vi "Mexa_One.vi"(0 "String 1 In":string, 1 "Connect":bool, 5 "connection ID 1 In":refnum<k5>, 7 "error out 1 In":errorcluster, 9 "connection ID 2 In":refnum<k16>, 11 "error out 2 In":errorcluster, 12 "Time In":i16, 13 "Test Loop":dbl) -> (3 "Emissions":dbl[](array[numeric]), 4 "String 1 Out":string, 6 "connection ID 1 Out":refnum<k5>, 8 "error 1 out":errorcluster, 10 "connection ID 2 Out":refnum<k16>, 14 "Time Out":i16, 15 "error 2 out":errorcluster)   [LabVIEW 2014]
panel:
  in  "stop":bool
  out "Array out":dbl[](array[numeric])
  in  "stop TCP 2":bool
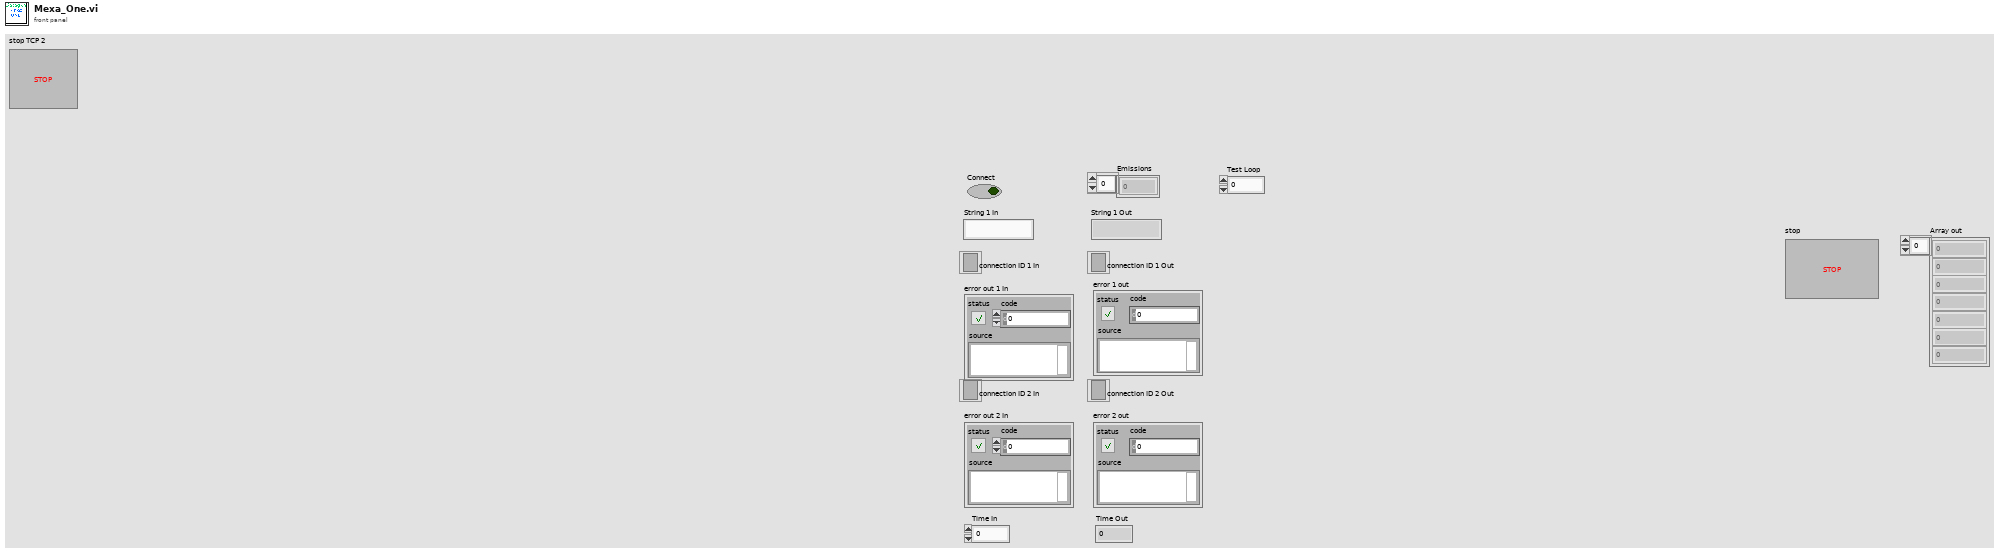
[diagram p1: front panel]
types:
  T1 = cluster{"status":bool, "code":bool, "source":bool}
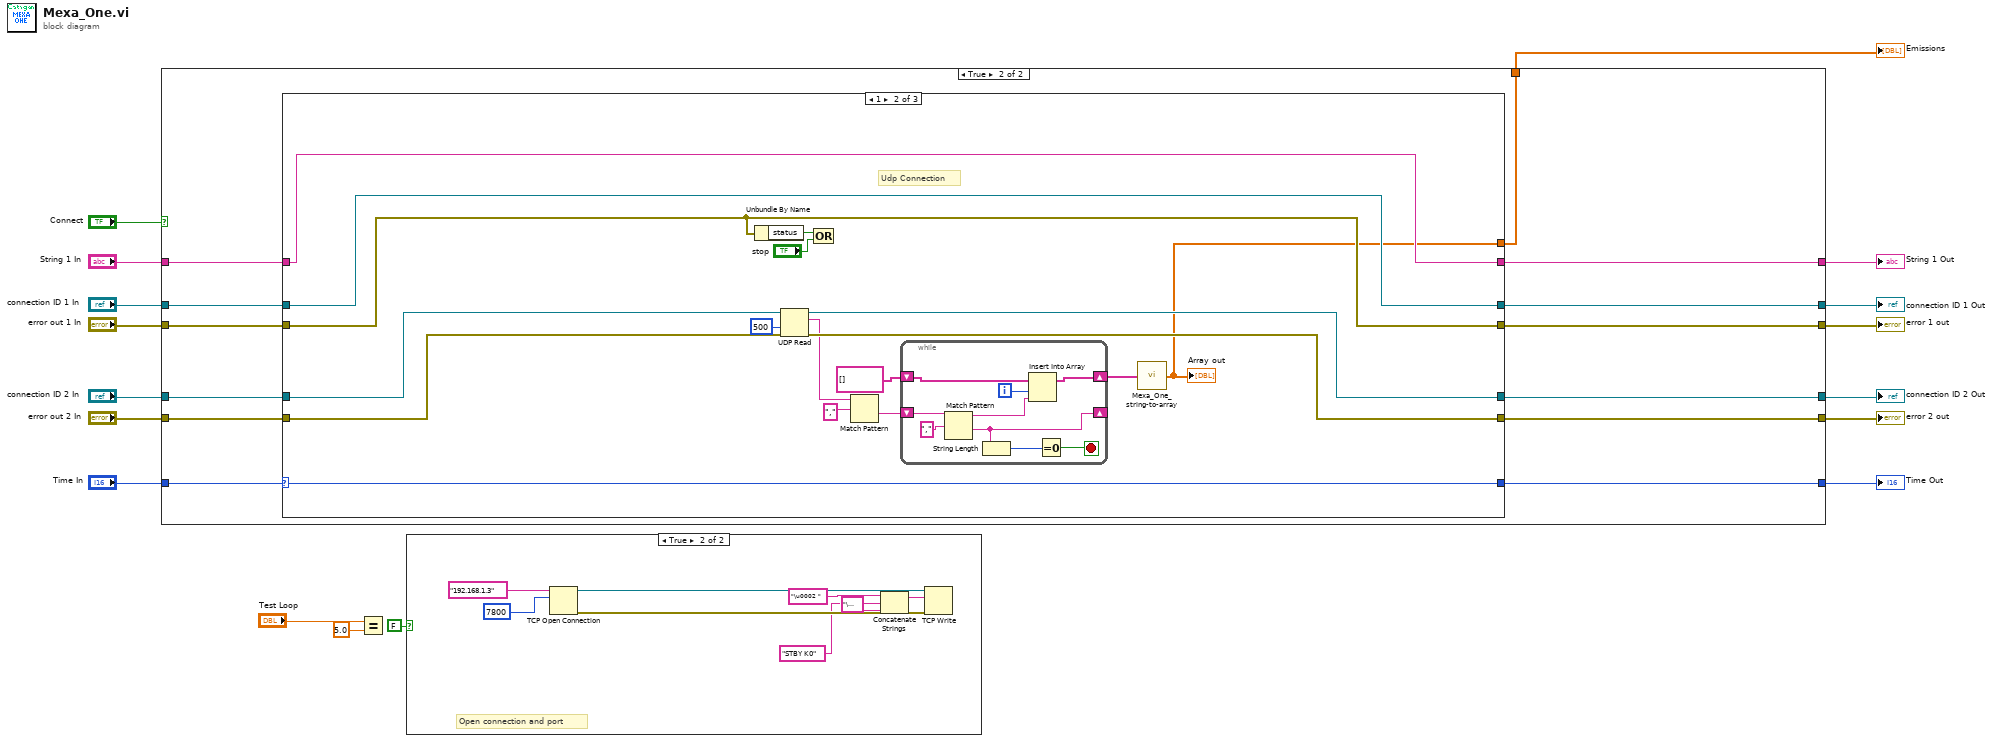
[diagram p0: block diagram]
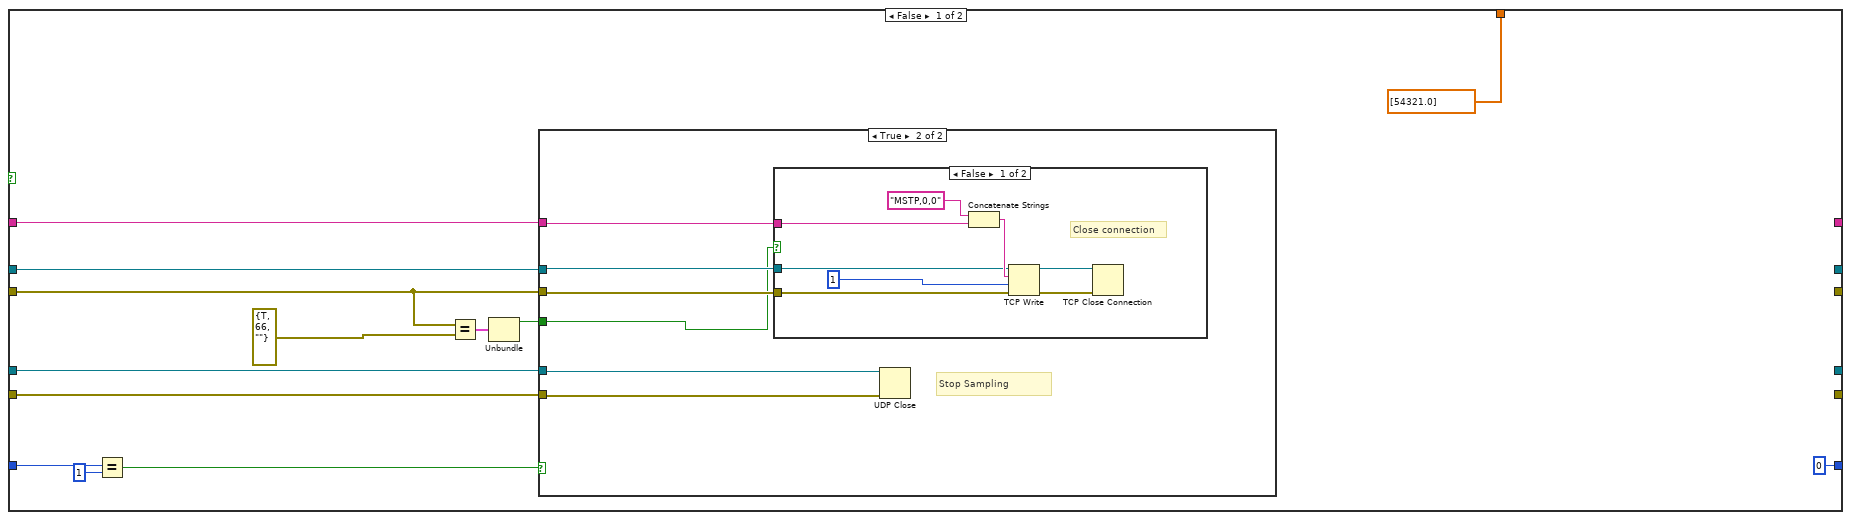
[diagram p3: hidden frame]
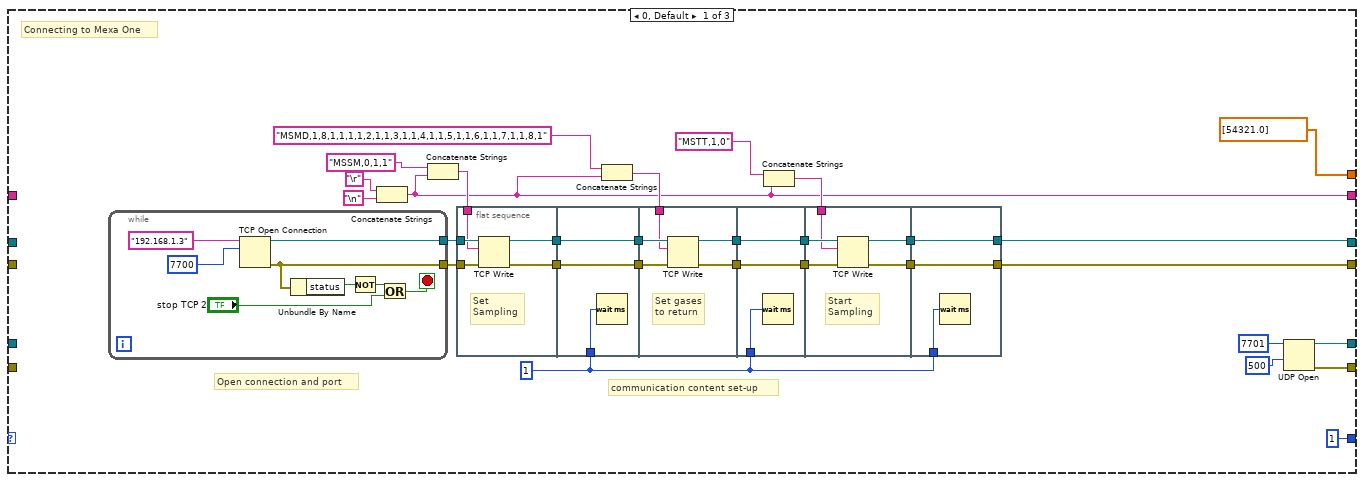
[diagram p6: hidden frame]
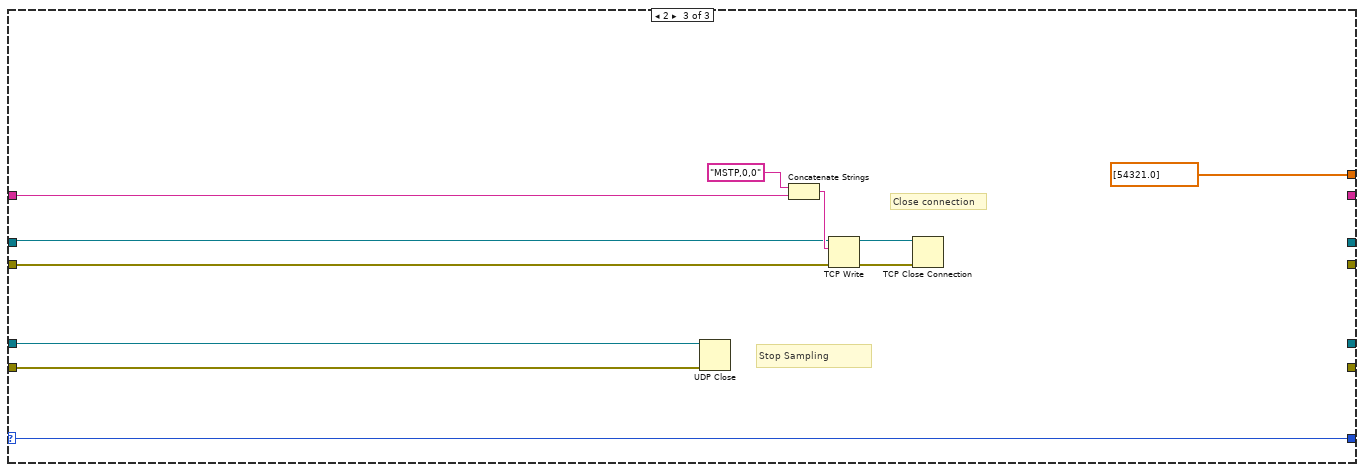
[diagram p7: hidden frame]
diagram:
  n1 = case shown="True" "Connect" {
    tunnel: [dbl[] [54321.0] w57] -> w4
    tunnel: [_ w56] -> w6
    tunnel: [_ w55] -> w7
    tunnel: "connection ID 1 In" -> [w24 w54]
    tunnel: "error out 1 In" -> [w21 w53]
    tunnel: [_ w52] -> w5
    tunnel: "String 1 In" -> [w25 w51]
    tunnel: [_ w50] -> w8
    tunnel: [_ w49] -> w9
    tunnel: "connection ID 2 In" -> [w23 w48]
    tunnel: "error out 2 In" -> [w22 w47]
    tunnel: "Time In" -> [w28 w46]
    tunnel: [i16 0 ("MKS 2") w45] -> w10
    frame False {
      n2 = Equal?(x=w28, y=i16 1) -> (x = y?=w26:bool)
      n3 = Equal?(x=w21, y=errorcluster {"status"=TRUE, "code"=66, "source"=""}) -> (x = y?=w19:T1)
      n4 = Unbundle(w19) -> ("status"=w18:bool)  [unwired: 2 out]
      n5 = case shown="True" w26 {
        tunnel: w25 -> [_ w36]
        tunnel: w24 -> [_ w32]
        tunnel: w21 -> [_ w33]
        tunnel: w23 -> [_ w35]
        tunnel: w22 -> [_ w34]
        tunnel: w18 -> [_ w31]
        frame False {
        }
        frame True {
          # "Stop Sampling"
          n6 = case shown="False" w31 {
            tunnel: w36 -> [w40 _]
            tunnel: w33 -> [w39 _]
            tunnel: w32 -> [w38 _]
            frame False {
              # "Close connection"
              n7 = Concatenate Strings("MSTP,0,0" ("string"), w40) -> (w41:string)
              n8 = TCP Write(connection ID=w38, data in=w41, error in (no error)=w39, 9:1 ("timeout ms (25000)")) -> (connection ID out=w43:refnum<k5>, error out=w44:errorcluster)  [unwired: 1 out]
              n9 = TCP Close Connection(connection ID=w43, error in (no error)=w44) -> ()  [unwired: 1 in, 2 out]
            }
            frame True {
            }
          }
          n10 = UDP Close(connection ID=w35, 8:w34) -> ()  [unwired: 2 out]
        }
      }
    }
    frame True {
      n11 = case shown="1" w46 {
        selector: w46 -> [_ w122 w147]
        tunnel: [dbl[] [54321.0] w120 dbl[] [54321.0]] -> w57
        tunnel: [w65 w135 _] -> w56
        tunnel: [w64 w134 _] -> w55
        tunnel: w54 -> [_ w135 w152]
        tunnel: w53 -> [_ w134 w151]
        tunnel: [w63 w136 _] -> w52
        tunnel: w51 -> [_ w136 w146]
        tunnel: [w60 w131 _] -> w50
        tunnel: [w59 w130 _] -> w49
        tunnel: w48 -> [_ w133 w150]
        tunnel: w47 -> [_ w132 w149]
        tunnel: [i16 1 ("MKS 2") w122 w147] -> w45
        frame 0, Default {
          w66 = 1
          # "Open connection and port"
          # "communication content set-up"
          # "Connecting to Mexa One"
          n12 = while {
            tunnel: [w116] -> w76
            tunnel: [w115] -> w75
            stop <- w112 stop-if-true
            n13 = TCP Open Connection(address="192.168.1.3", remote port or service name=u16 7700) -> (connection ID=w116:refnum<k5>, error out=w115:errorcluster)  [unwired: 3 in]
            n14 = Unbundle By Name(w115) -> ("status"=w117:bool)
            n15 = Not(x=w117) -> (.not. x?=w113:bool)
            n16 = Or(x=w113, y="stop TCP 2") -> (x .or. y?=w112:bool)
          }
          n17 = Concatenate Strings("\r", "\n") -> (w63:string)
          n18 = Concatenate Strings("MSSM,0,1,1" ("data in"), w63) -> (w71:string)
          n19 = flat-sequence {
            tunnel: w76 -> [w92]
            tunnel: w75 -> [w91]
            tunnel: w71 -> [w90]
            tunnel: [w89] -> w86
            tunnel: [w88] -> w85
            tunnel: w86 -> [w95]
            tunnel: w85 -> [w94]
            tunnel: w66 -> [w93]
            tunnel: [w95] -> w84
            tunnel: [w94] -> w83
            tunnel: w84 -> [w99]
            tunnel: w83 -> [w100]
            tunnel: w68 -> [w98]
            tunnel: [w96] -> w82
            tunnel: [w97] -> w81
            tunnel: w82 -> [w103]
            tunnel: w81 -> [w102]
            tunnel: w66 -> [w101]
            tunnel: [w103] -> w80
            tunnel: [w102] -> w79
            tunnel: w80 -> [w107]
            tunnel: w79 -> [w108]
            tunnel: w67 -> [w104]
            tunnel: [w106] -> w78
            tunnel: [w105] -> w77
            tunnel: [w110] -> w65
            tunnel: [w111] -> w64
            tunnel: w78 -> [w111]
            tunnel: w77 -> [w110]
            tunnel: w66 -> [w109]
            frame #0 {
              # "Set \nSampling"
              n20 = TCP Write(connection ID=w92, data in=w90, error in (no error)=w91) -> (connection ID out=w88:refnum<k5>, error out=w89:errorcluster)  [unwired: 1 in, 1 out]
            }
            frame #1 {
              n21 = Wait (ms)(milliseconds to wait=w93) -> ()  [unwired: 1 out]
            }
            frame #2 {
              # "Set gases\nto return"
              n22 = TCP Write(connection ID=w100, data in=w98, error in (no error)=w99) -> (connection ID out=w97:refnum<k5>, error out=w96:errorcluster)  [unwired: 1 in, 1 out]
            }
            frame #3 {
              n23 = Wait (ms)(milliseconds to wait=w101) -> ()  [unwired: 1 out]
            }
            frame #4 {
              # "Start\nSampling"
              n24 = TCP Write(connection ID=w108, data in=w104, error in (no error)=w107) -> (connection ID out=w105:refnum<k5>, error out=w106:errorcluster)  [unwired: 1 in, 1 out]
            }
            frame #5 {
              n25 = Wait (ms)(milliseconds to wait=w109) -> ()  [unwired: 1 out]
            }
          }
          n26 = Concatenate Strings("MSMD,1,8,1,1,1,1,2,1,1,3,1,1,4,1,1,5,1,1,6,1,1,7,1,1,8,1" ("data in"), w63) -> (w68:string)
          n27 = Concatenate Strings("MSTT,1,0" ("string"), w63) -> (w67:string)
          n28 = UDP Open(9:500 ("timeout ms (25000)"), 11:u16 7701 ("port")) -> (port=w60:refnum<k16>, 0:w59:errorcluster)  [unwired: 3 in, 1 out]
        }
        frame 1 {
          # "Udp Connection"
          n29 = Unbundle By Name(w134) -> ("status"=w128:bool)
          n30 = UDP Read(connection ID=w133, timeout ms (25000)=500, 8:w132) -> (data out=w124:string, error out=w130:errorcluster, 3:w131:refnum<k16>)  [unwired: 1 in, 2 out]
          n31 = Compound Arithmetic op=OR(w128, "stop") -> ()  [unwired: 1 out]
          n32 = Match Pattern(string=w124, regular expression="," ("search string/char (-)")) -> (after substring=w125:string)  [unwired: 1 in, 3 out]
          n33 = while {
            shift-right: [w140] -> w121
            shift-left: string[] [] -> [w141]
            shift-right: [w139] -> _
            shift-left: w125 -> [w143]
            i -> [w145]
            stop <- w138 stop-if-true
            n34 = Match Pattern(string=w143, regular expression="," ("search string/char (-)")) -> (before substring=w142:string, after substring=w139:string)  [unwired: 1 in, 2 out]
            n35 = String Length(string=w139) -> (length=w137:i32)
            n36 = Insert Into Array(array=w141, index=w145, new element=w142) -> (w140:string[])
            n37 = Equal To 0?(x=w137) -> (x = 0?=w138:bool)
          }
          n38 = call "Mexa_One_string-to-array.vi"("Array in"=w121) -> ("Array out"=w120:dbl[])  [unwired: 4 in]
          "Array out" <- w120
        }
        frame 2 {
          # "Close connection"
          # "Stop Sampling"
          n39 = UDP Close(connection ID=w150, 8:w149) -> ()  [unwired: 2 out]
          n40 = Concatenate Strings("MSTP,0,0" ("string"), w146) -> (w153:string)
          n41 = TCP Write(connection ID=w152, data in=w153, error in (no error)=w151) -> (connection ID out=w155:refnum<k5>, error out=w156:errorcluster)  [unwired: 1 in, 1 out]
          n42 = TCP Close Connection(connection ID=w155, error in (no error)=w156) -> ()  [unwired: 1 in, 2 out]
        }
      }
    }
  }
  "Time Out" <- w10
  "error 2 out" <- w9
  "connection ID 2 Out" <- w8
  "error 1 out" <- w7
  "connection ID 1 Out" <- w6
  "String 1 Out" <- w5
  "Emissions" <- w4
  n43 = Equal?(x="Test Loop", y=5.0) -> ()  [unwired: 1 out]
  n44 = case shown="True" FALSE {
    frame False {
    }
    frame True {
      # "Open connection and port"
      n45 = TCP Open Connection(address="192.168.1.3", remote port or service name=u16 7800) -> (connection ID=w164:refnum<k5>, error out=w163:errorcluster)  [unwired: 3 in]
      n46 = Concatenate Strings("\u0002 " ("string"), "STBY K0" ("string"), "\u0003" ("string")) -> (w160:string)
      n47 = TCP Write(connection ID=w164, data in=w160, error in (no error)=w163) -> ()  [unwired: 1 in, 3 out]
    }
  }
